vi "soilwave_sinusodial.vi"(1 "Depth (m)":dbl, 2 "Thermal diffusivity (m2 s-1)":dbl=0.8, 3 "Time (s)":dbl, 4 "Period of wave (s)":dbl=86400.0, 5 "Surface temperature amplitude (K)":dbl=10.0, 6 "Mean surface temperature (¼C)":dbl=15.0) -> (0 "Soil temperature (z,t) (¼C)":dbl)   [LabVIEW 2012]
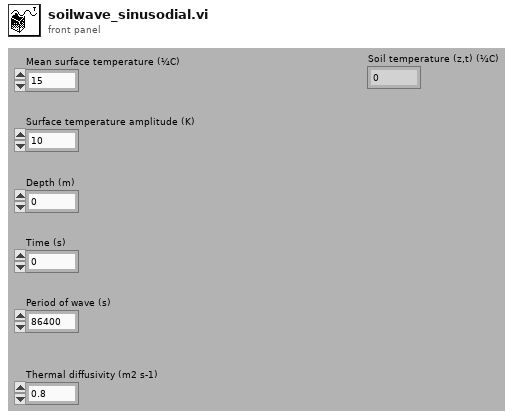
[diagram p1: front panel]
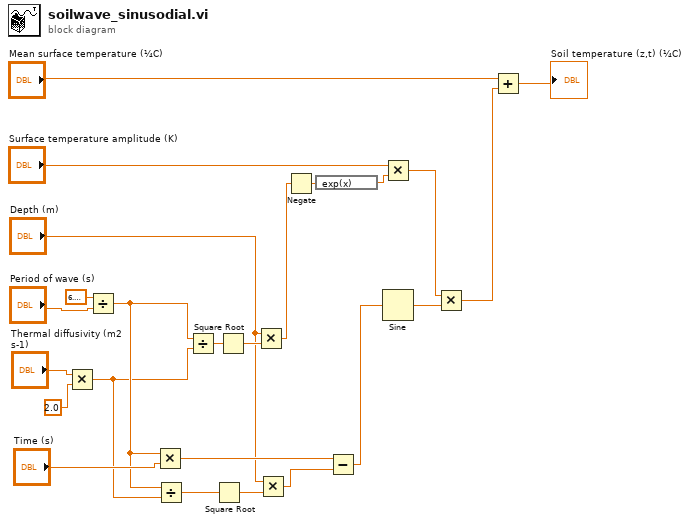
[diagram p0: block diagram]
diagram:
  n1 = Multiply(x="Thermal diffusivity (m2 s-1)", y=2.0) -> (x*y=w5:dbl)
  n2 = Divide(x=6.283185307179586, y="Period of wave (s)") -> (x/y=w6:dbl)
  n3 = Multiply(x=w6, y="Time (s)") -> (x*y=w8:dbl)
  n4 = Divide(x=w6, y=w5) -> (x/y=w7:dbl)
  n5 = Divide(x=w6, y=w5) -> (x/y=w15:dbl)
  n6 = Square Root(x=w7) -> (sqrt(x)=w4:dbl)
  n7 = Square Root(x=w15) -> (sqrt(x)=w14:dbl)
  n8 = Multiply(x="Depth (m)", y=w14) -> (x*y=w13:dbl)
  n9 = Multiply(x="Depth (m)", y=w4) -> (x*y=w2:dbl)
  n10 = Negate(x=w13) -> (-x=w20:dbl)
  n11 = expression code="exp(x)"(w20) -> (w21:dbl)
  n12 = Subtract(x=w8, y=w2) -> (x-y=w1:dbl)
  n13 = Multiply(x="Surface temperature amplitude (K)", y=w21) -> (x*y=w11:dbl)
  n14 = Sine(x=w1) -> (sin(x)=w10:dbl)
  n15 = Multiply(x=w11, y=w10) -> (x*y=w12:dbl)
  n16 = Add(x="Mean surface temperature (¼C)", y=w12) -> (x+y=→"Soil temperature (z,t) (¼C)":dbl)
